vi "读取反控数据解析(子VI).vi"(6 "数据":string, 7 "命令编码CN":string) -> (2 "设置超时时间/min":i32=1, 3 "反控命令错误？":bool)   [LabVIEW 2016, in "数据传输系统.lvlib"]
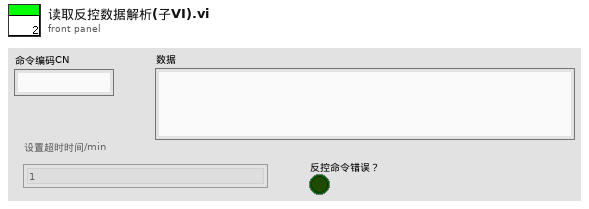
[diagram p1: front panel]
types:
  T1 = enum16{"初始化", "打开连接", "表格比对", "发送数据", "读取数据", "数据处理"}
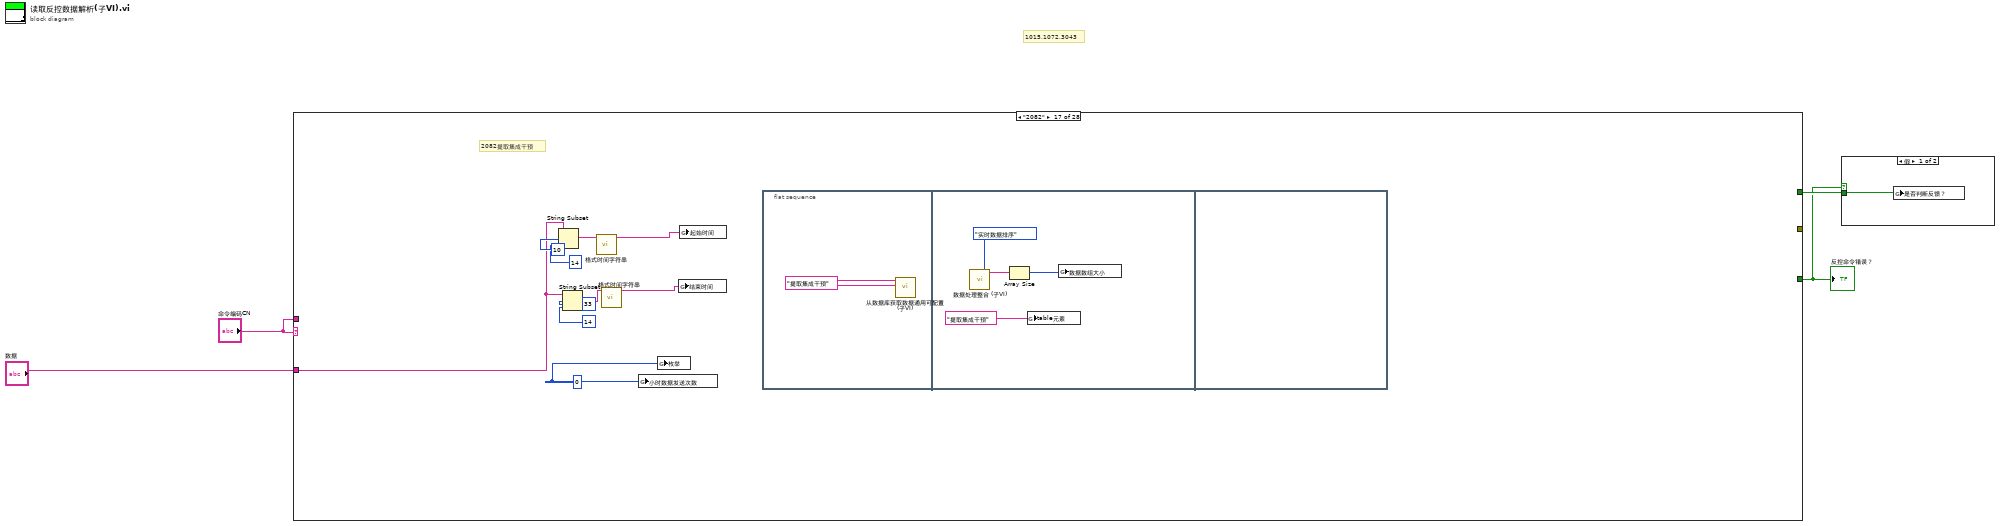
[diagram p0: block diagram]
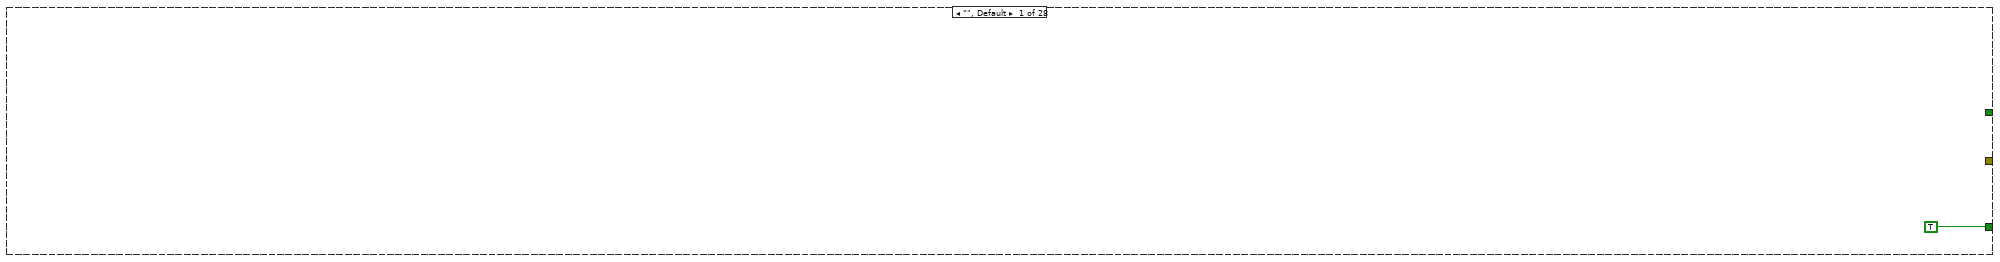
[diagram p3: hidden frame]
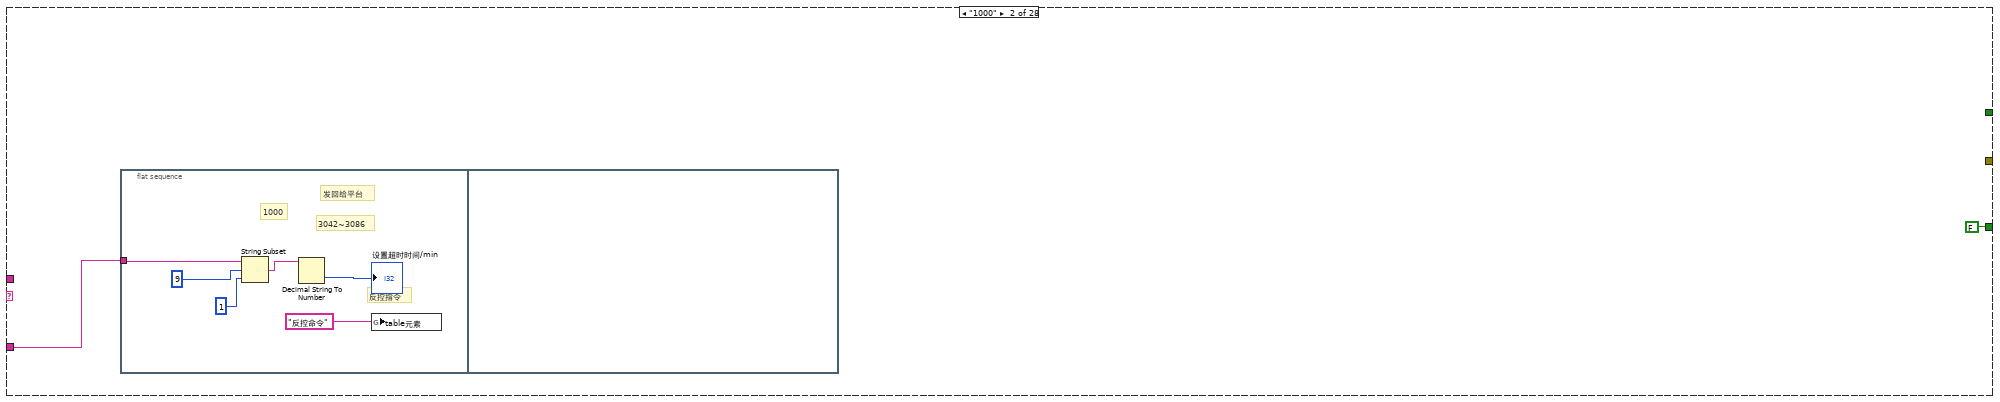
[diagram p4: hidden frame]
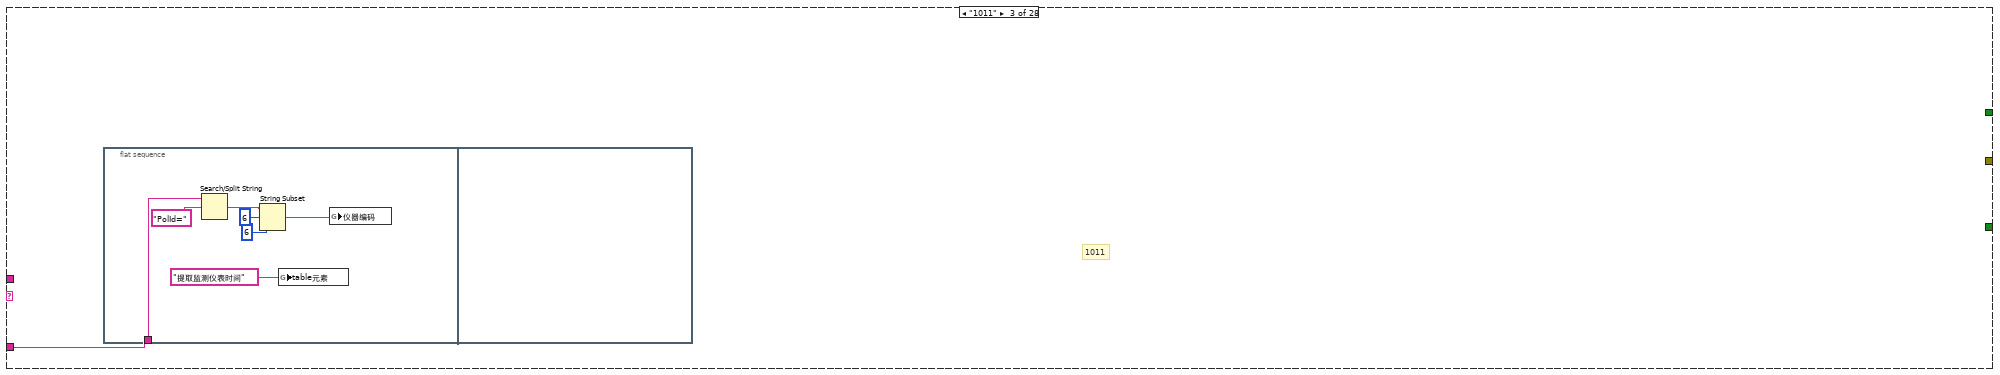
[diagram p5: hidden frame]
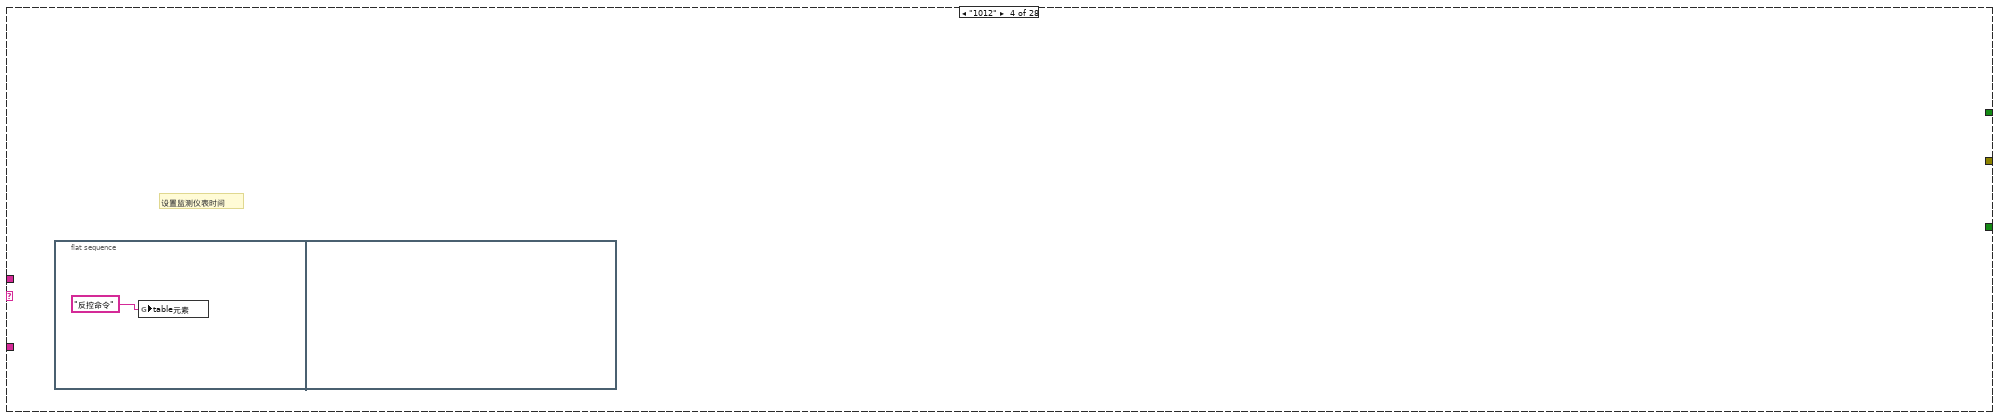
[diagram p6: hidden frame]
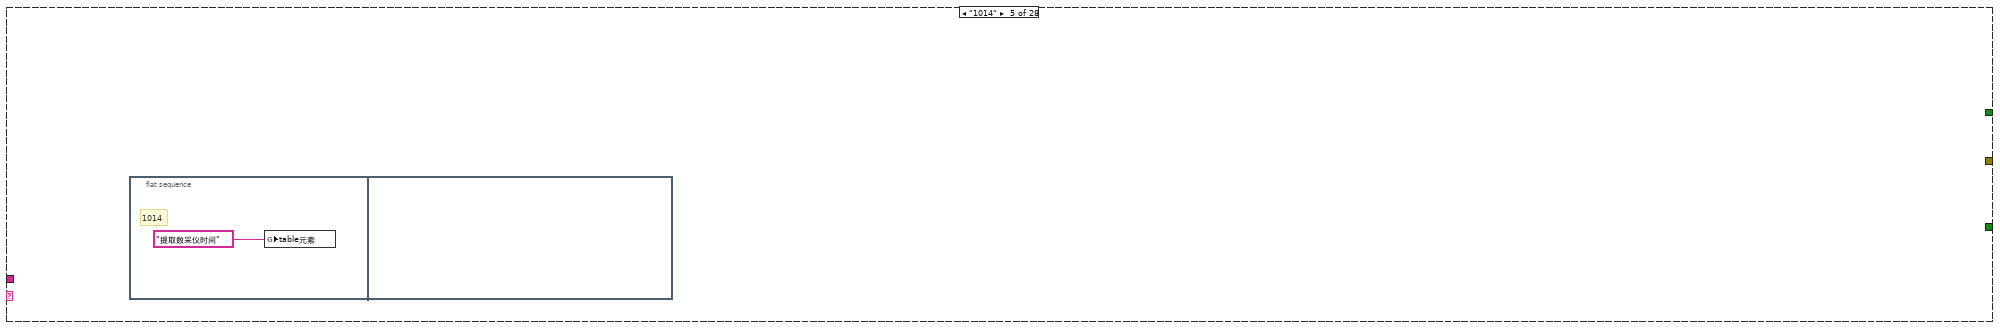
[diagram p7: hidden frame]
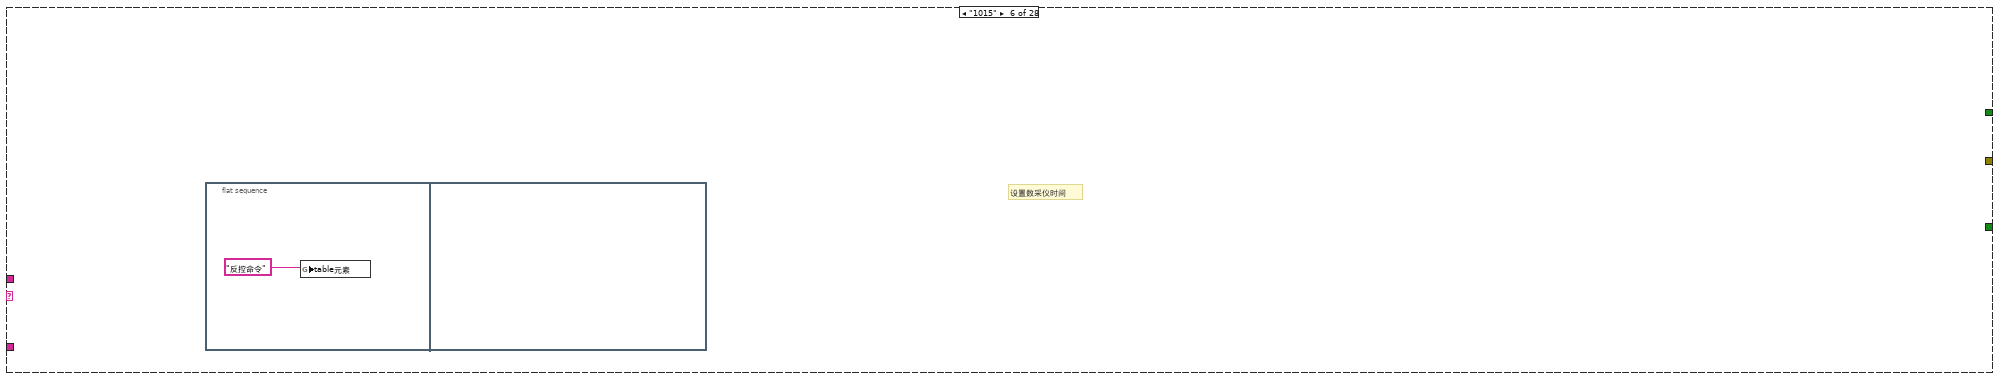
[diagram p8: hidden frame]
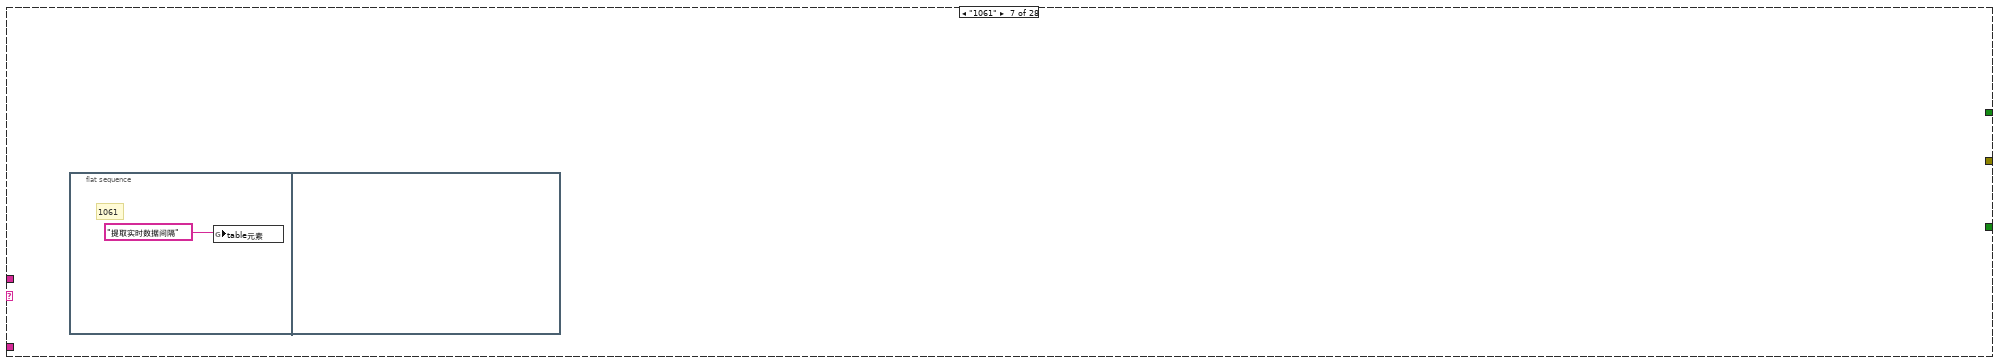
[diagram p9: hidden frame]
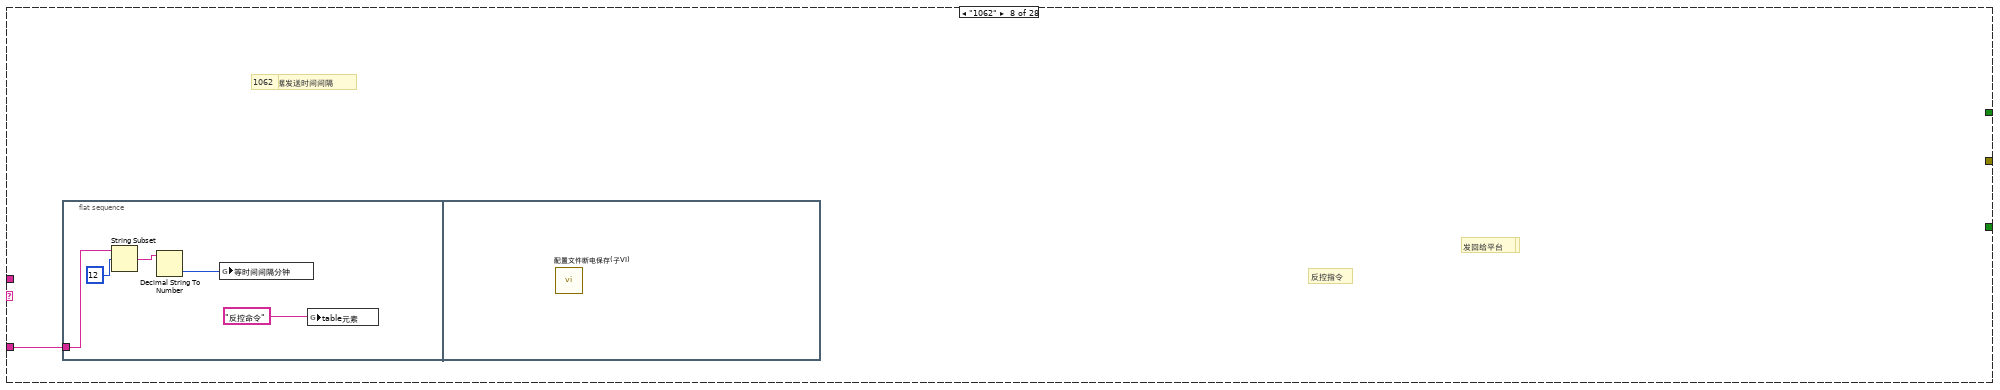
[diagram p10: hidden frame]
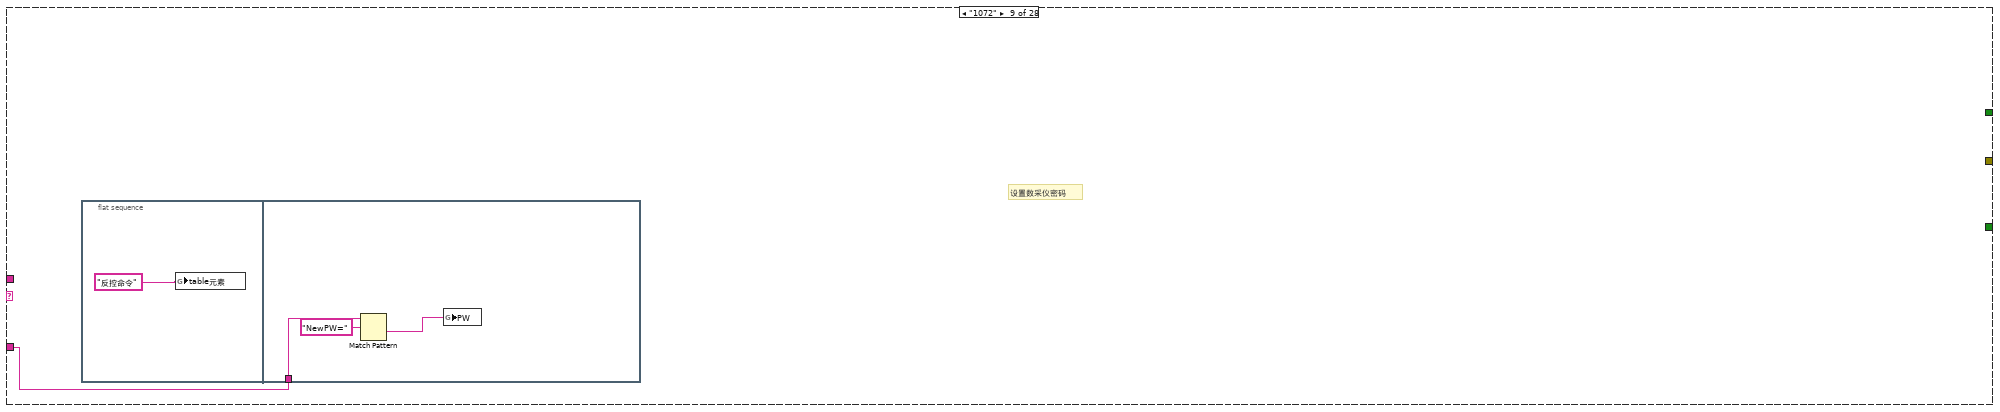
[diagram p11: hidden frame]
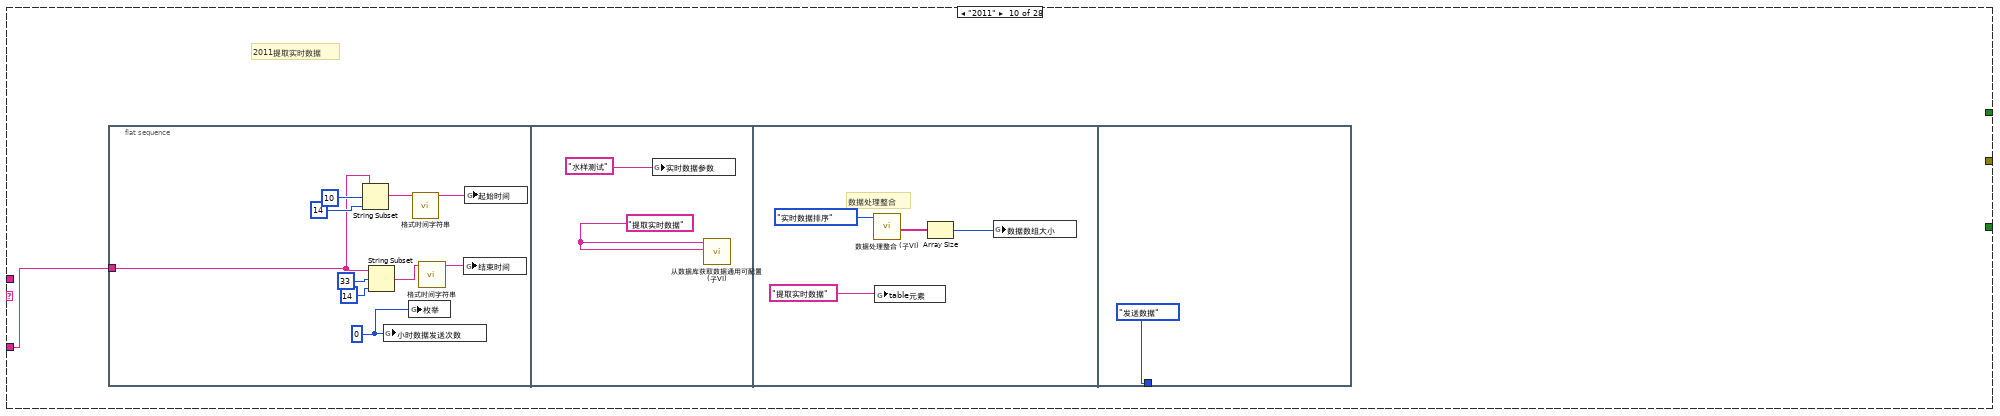
[diagram p12: hidden frame]
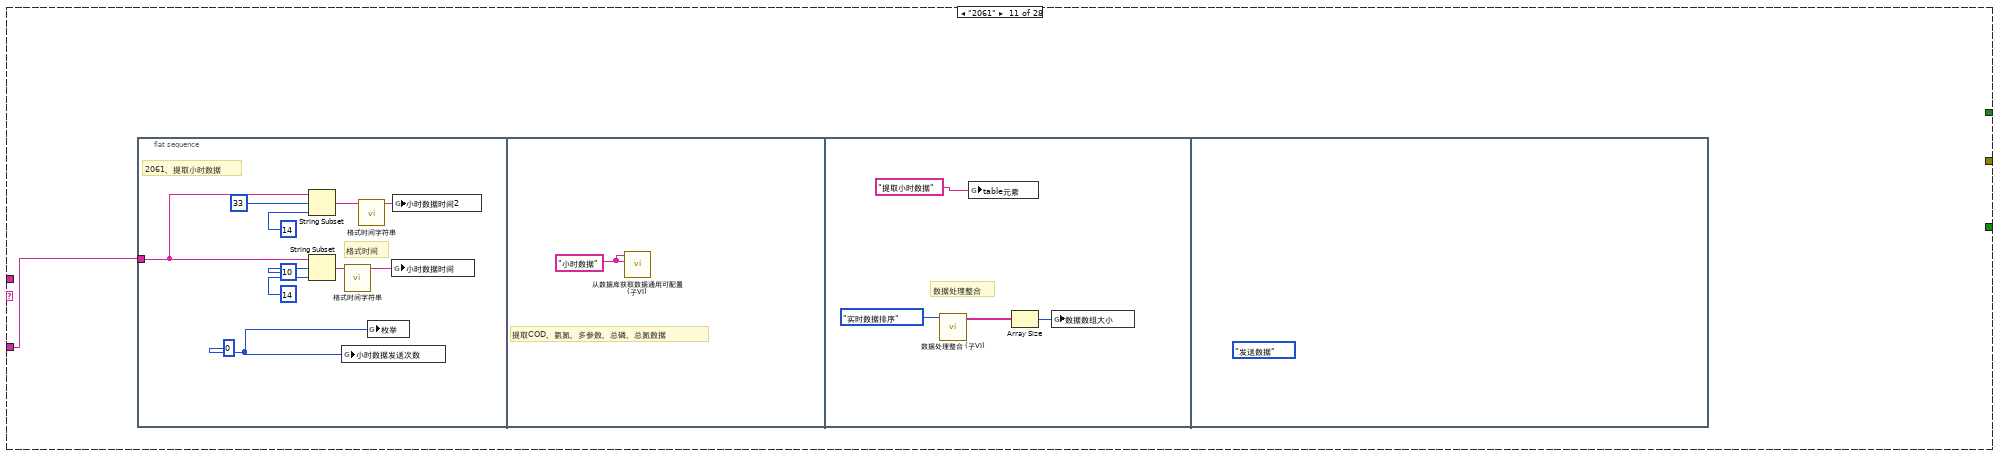
[diagram p13: hidden frame]
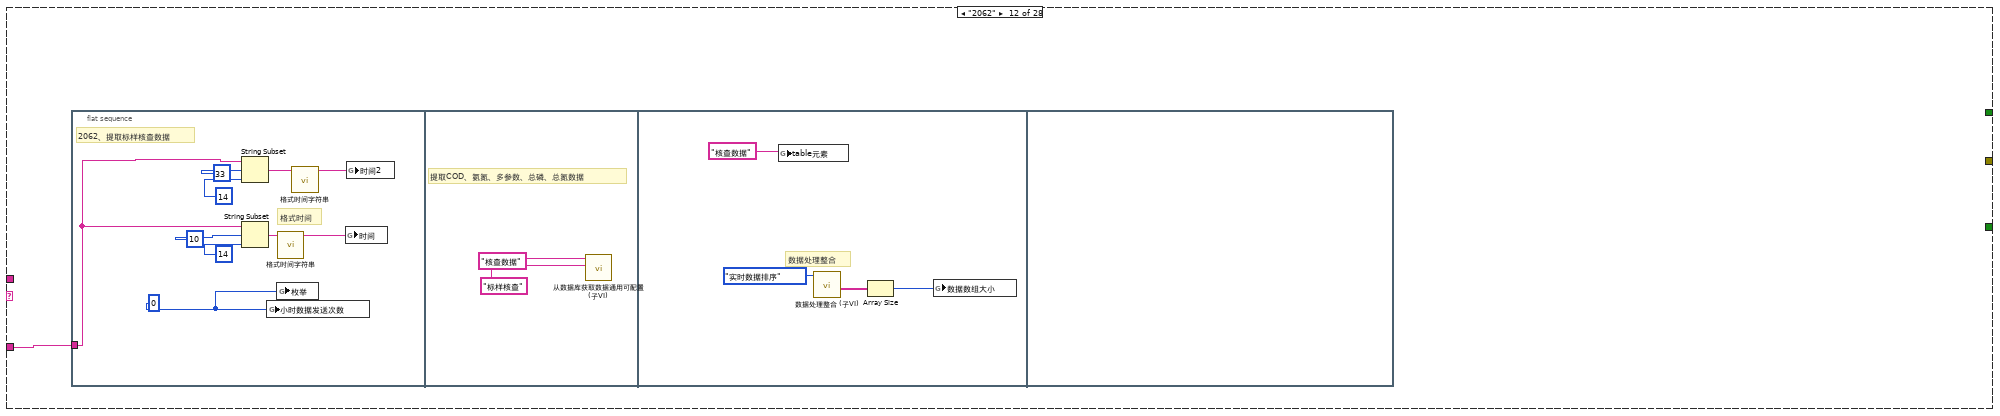
[diagram p14: hidden frame]
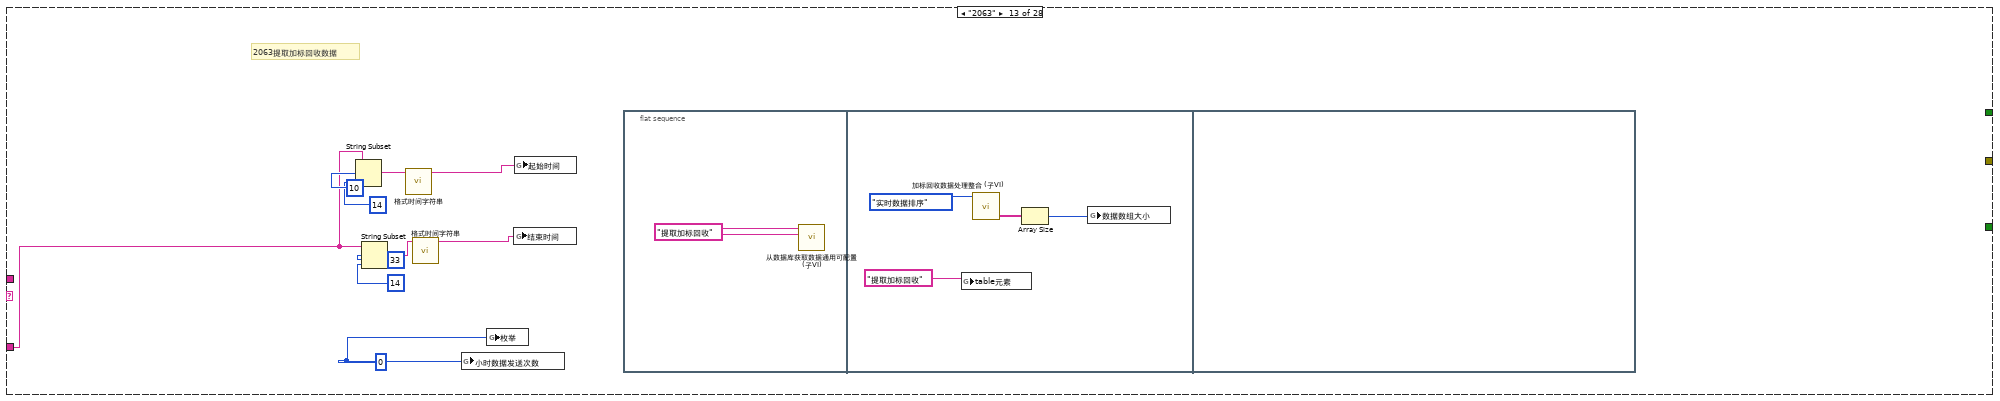
[diagram p15: hidden frame]
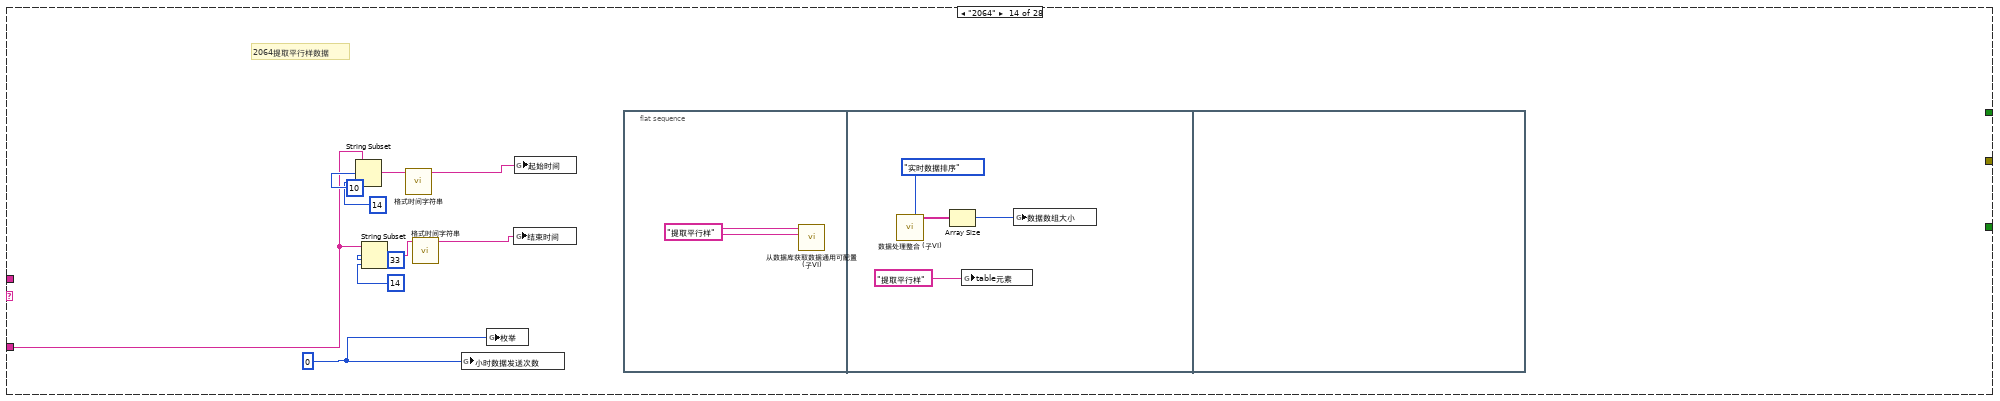
[diagram p16: hidden frame]
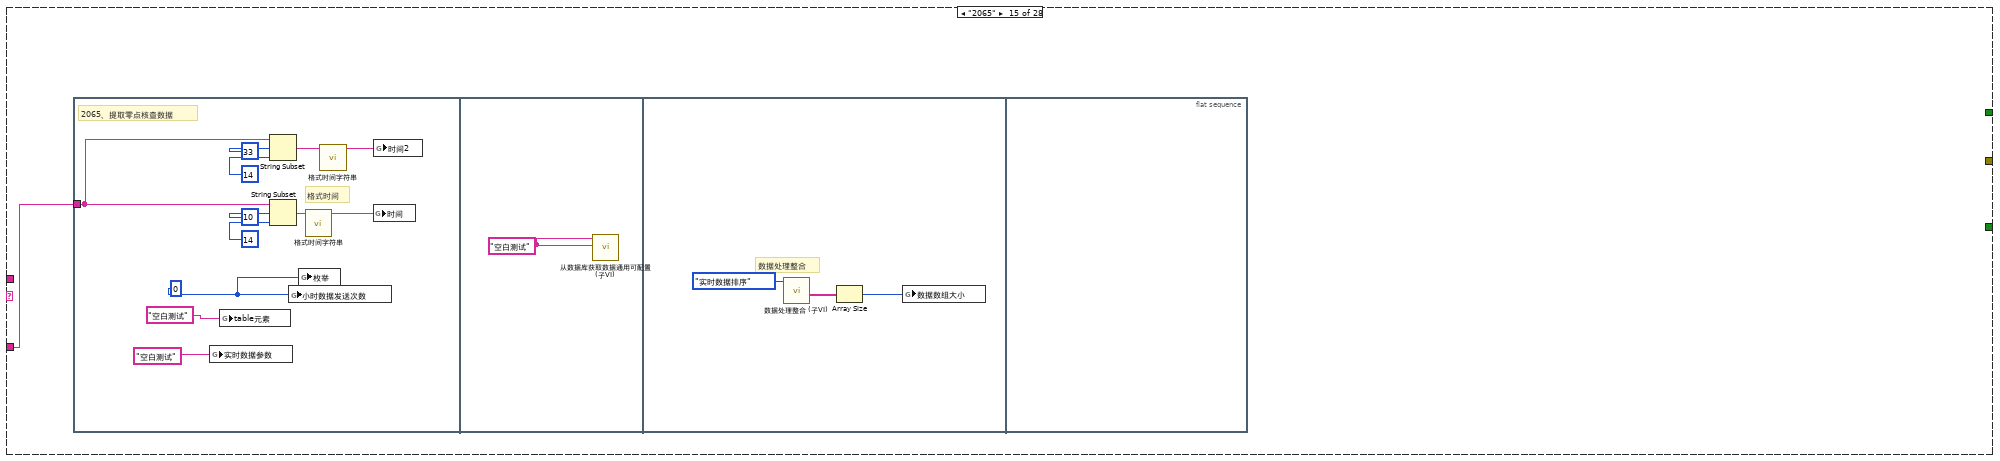
[diagram p17: hidden frame]
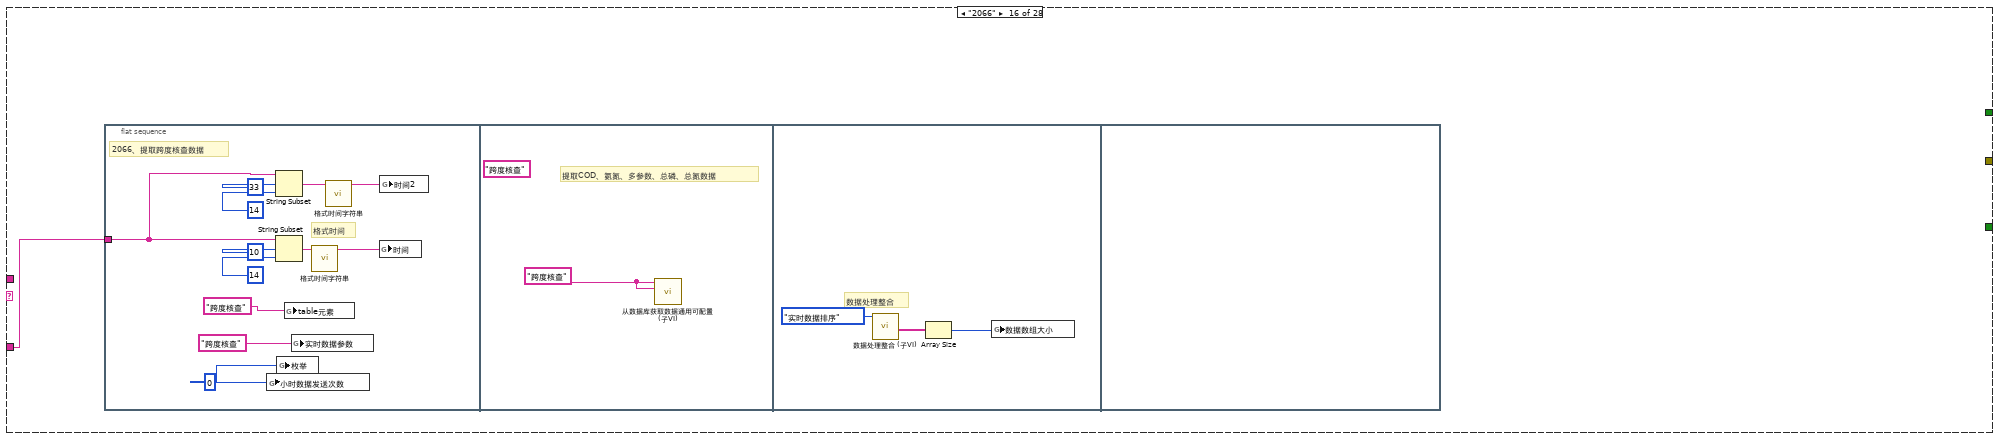
[diagram p18: hidden frame]
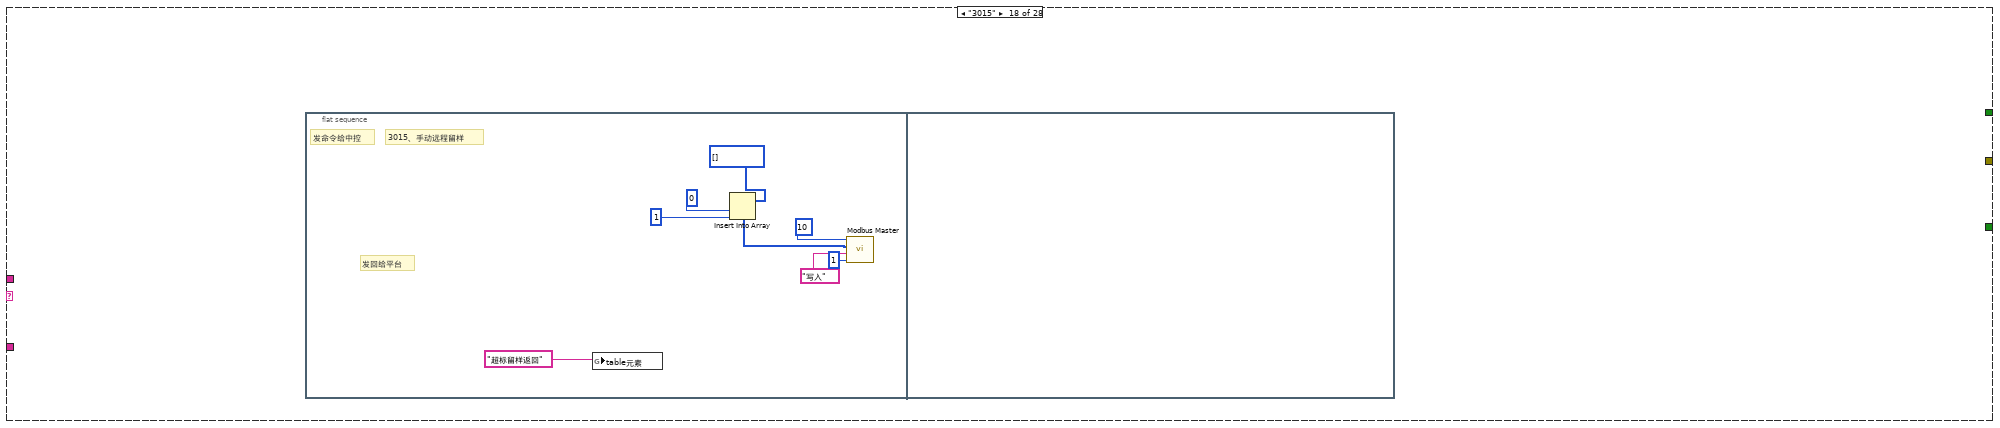
[diagram p19: hidden frame]
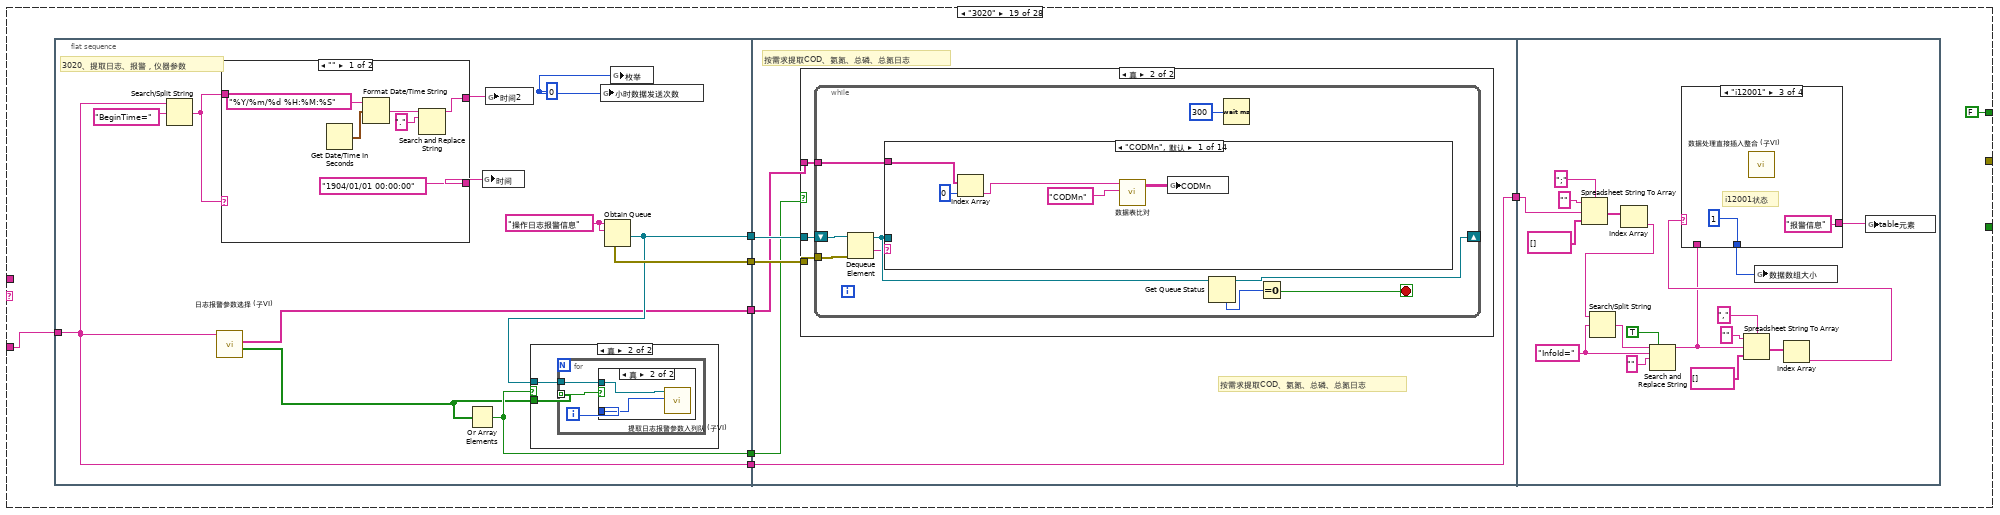
[diagram p20: hidden frame]
diagram:
  # "1015,1072,3043"
  n1 = case shown="\"2082\"" "命令编码CN" {
    tunnel: "命令编码CN" -> [_ _ _ _ _ _ _ _ _ _ _ _ _ _ _ _ _ _ _ _ _ _ _ _ _ _ _ w475]
    tunnel: "数据" -> [_ w7 w14 _ _ _ _ w26 w32 w37 w55 w71 w88 w103 w118 w135 w152 _ w178 w334 _ _ w412 _ _ _ w456 w472]
    tunnel: [_ _ _ _ _ _ _ _ _ _ _ _ _ _ _ _ _ _ _ _ _ _ _ _ _ _ _ w470] -> _
    tunnel: [TRUE FALSE _ _ _ _ _ _ _ _ _ _ _ _ _ _ _ _ _ _ _ _ _ _ _ _ _ _] -> w1
    tunnel: [_ _ _ _ _ _ _ _ _ _ _ _ _ _ _ _ _ _ FALSE ("是否判断反馈？") TRUE ("是否判断反馈？") _ _ TRUE ("是否判断反馈？") _ TRUE ("是否判断反馈？") TRUE ("是否判断反馈？") _ TRUE ("是否判断反馈？")] -> w2
    frame "", Default {
    }
    frame "1000" {
      n2 = flat-sequence {
        tunnel: w7 -> [w9]
        frame #0 {
          # "发回给平台"
          # "3042~3086"
          # "反控指令"
          # "1000"
          n3 = String Subset(string=w9, offset (0)=9 ("偏移量(0)"), length (rest)=1 ("长度（剩余）")) -> (substring=w11:string)
          n4 = Decimal String To Number(string=w11) -> (number=→"设置超时时间/min":i32)  [unwired: 2 in, 1 out]
          n5 = global write "全局1.vi" "table元素"("反控命令" ("新元素/子数组")) -> ()
        }
        frame #1 {
        }
      }
    }
    frame "1011" {
      # "1011"
      n6 = flat-sequence {
        tunnel: w14 -> [w16]
        frame #0 {
          n7 = Search/Split String(string=w16, search string/char (-)="PolId=" ("搜索字符串/字符(-)")) -> (match + rest of string=w20:string)  [unwired: 1 in, 2 out]
          n8 = String Subset(string=w20, offset (0)=6 ("偏移量(0)"), length (rest)=6 ("长度（剩余）")) -> (substring=w17:string)
          n9 = global write "全局1.vi" "table元素"("提取监测仪表时间") -> ()
          n10 = global write "全局 提取仪器参数.vi" "仪器编码"(w17) -> ()
        }
        frame #1 {
        }
      }
    }
    frame "1012" {
      # "设置监测仪表时间"
      n11 = flat-sequence {
        frame #0 {
          n12 = global write "全局1.vi" "table元素"("反控命令" ("新元素/子数组")) -> ()
        }
        frame #1 {
        }
      }
    }
    frame "1014" {
      n13 = flat-sequence {
        frame #0 {
          # "1014"
          n14 = global write "全局1.vi" "table元素"("提取数采仪时间") -> ()
        }
        frame #1 {
        }
      }
    }
    frame "1015" {
      # "设置数采仪时间"
      n15 = flat-sequence {
        frame #0 {
          n16 = global write "全局1.vi" "table元素"("反控命令" ("新元素/子数组")) -> ()
        }
        frame #1 {
        }
      }
    }
    frame "1061" {
      n17 = flat-sequence {
        frame #0 {
          # "1061"
          n18 = global write "全局1.vi" "table元素"("提取实时数据间隔") -> ()
        }
        frame #1 {
        }
      }
    }
    frame "1062" {
      # "发回给平台"
      # "反控指令"
      # "3042~3086"
      # "设置数据发送时间间隔"
      # "1062"
      n19 = flat-sequence {
        tunnel: w26 -> [w29]
        frame #0 {
          n20 = String Subset(string=w29, offset (0)=12 ("偏移量(0)")) -> (substring=w30:string)  [unwired: 1 in]
          n21 = Decimal String To Number(string=w30) -> (number=w27:i32)  [unwired: 2 in, 1 out]
          n22 = global write "断电保存全局.vi" "等时间间隔分钟"(w27) -> ()
          n23 = global write "全局1.vi" "table元素"("反控命令" ("新元素/子数组")) -> ()
        }
        frame #1 {
          n24 = call "配置文件断电保存(子VI).vi"() -> ()  [unwired: 12 in]
        }
      }
    }
    frame "1072" {
      # "设置数采仪密码"
      n25 = flat-sequence {
        tunnel: w32 -> [w36]
        frame #0 {
          n26 = global write "全局1.vi" "table元素"("反控命令" ("新元素/子数组")) -> ()
        }
        frame #1 {
          n27 = Match Pattern(string=w36, regular expression="NewPW=" ("正则表达式")) -> (after substring=w34:string)  [unwired: 1 in, 3 out]
          n28 = global write "断电保存全局.vi" "PW"(w34) -> ()
        }
      }
    }
    frame "2011" {
      # "2011提取实时数据"
      n29 = flat-sequence {
        tunnel: w37 -> [w38]
        tunnel: [T1."发送数据" ("元素")] -> _
        frame #0 {
          w43 = 0 ("数值")
          n30 = String Subset(string=w38, offset (0)=10 ("偏移量(0)"), length (rest)=14 ("长度（剩余）")) -> (substring=w46:string)
          n31 = String Subset(string=w38, offset (0)=33 ("偏移量(0)"), length (rest)=14 ("长度（剩余）")) -> (substring=w44:string)
          n32 = global write "全局 小时数据发送次数.vi" "小时数据发送次数"(w43) -> ()
          n33 = global write "全局1.vi" "枚举"(w43) -> ()
          n34 = call "格式时间字符串.vi"("字符串"=w46) -> ("连接的字符串"=w47:string)  [unwired: 10 in]
          n35 = call "格式时间字符串.vi"("字符串"=w44) -> ("连接的字符串"=w45:string)  [unwired: 10 in]
          n36 = global write "起始时间.vi" "结束时间"(w45) -> ()
          n37 = global write "起始时间.vi" "起始时间"(w47) -> ()
        }
        frame #1 {
          w48 = "提取实时数据" ("新元素/子数组")
          n38 = global write "全局 实时数据参数.vi" "实时数据参数"("水样测试") -> ()
          n39 = call "从数据库获取数据通用可配置(子VI).vi"("table输入"=w48, "列队名（唯一）"=w48) -> ()  [unwired: 8 in, 2 out]
        }
        frame #2 {
          # "数据处理整合"
          n40 = call "数据处理整合 (子VI).vi"("枚举"=enum16{"实时数据排序", "小时数据排序"}."实时数据排序") -> ("已排序的数组"=w52:string[])  [unwired: 10 in]
          n41 = global write "全局1.vi" "table元素"("提取实时数据" ("新元素/子数组")) -> ()
          n42 = Array Size(array=w52) -> (size(s)=w53:i32)
          n43 = global write "全局 数据数组大小.vi" "数据数组大小"(w53) -> ()
        }
        frame #3 {
        }
      }
    }
    frame "2061" {
      n44 = flat-sequence {
        tunnel: w55 -> [w56]
        frame #0 {
          w57 = 0 ("数值")
          # "格式时间"
          # "2061、提取小时数据"
          n45 = String Subset(string=w56, offset (0)=33 ("偏移量(0)"), length (rest)=14 ("长度（剩余）")) -> (substring=w59:string)
          n46 = String Subset(string=w56, offset (0)=10 ("偏移量(0)"), length (rest)=14 ("长度（剩余）")) -> (substring=w60:string)
          n47 = global write "全局 小时数据发送次数.vi" "小时数据发送次数"(w57) -> ()
          n48 = call "格式时间字符串.vi"("字符串"=w60) -> ("连接的字符串"=w61:string)  [unwired: 10 in]
          n49 = call "格式时间字符串.vi"("字符串"=w59) -> ("连接的字符串"=w58:string)  [unwired: 10 in]
          n50 = global write "全局1.vi" "枚举"(w57) -> ()
          n51 = global write "全局 水样时间.vi" "小时数据时间"(w61) -> ()
          n52 = global write "全局 时间2.vi" "小时数据时间2"(w58) -> ()
        }
        frame #1 {
          w66 = "小时数据" ("名称（未命名）")
          # "提取COD、氨氮、多参数、总磷、总氮数据"
          n53 = call "从数据库获取数据通用可配置(子VI).vi"("table输入"=w66, "列队名（唯一）"=w66) -> ()  [unwired: 8 in, 2 out]
        }
        frame #2 {
          # "数据处理整合"
          n54 = call "数据处理整合 (子VI).vi"("枚举"=enum16{"实时数据排序", "小时数据排序"}."实时数据排序") -> ("已排序的数组"=w70:string[])  [unwired: 10 in]
          n55 = global write "全局1.vi" "table元素"("提取小时数据" ("新元素/子数组")) -> ()
          n56 = Array Size(array=w70) -> (size(s)=w69:i32)
          n57 = global write "全局 数据数组大小.vi" "数据数组大小"(w69) -> ()
        }
        frame #3 {
          (unwired) T1."发送数据" ("元素")
        }
      }
    }
    frame "2062" {
      n58 = flat-sequence {
        tunnel: w71 -> [w72]
        frame #0 {
          w73 = 0 ("数值")
          # "格式时间"
          # "2062、提取标样核查数据"
          n59 = String Subset(string=w72, offset (0)=33 ("偏移量(0)"), length (rest)=14 ("长度（剩余）")) -> (substring=w75:string)
          n60 = String Subset(string=w72, offset (0)=10 ("偏移量(0)"), length (rest)=14 ("长度（剩余）")) -> (substring=w76:string)
          n61 = global write "全局 小时数据发送次数.vi" "小时数据发送次数"(w73) -> ()
          n62 = global write "全局1.vi" "枚举"(w73) -> ()
          n63 = call "格式时间字符串.vi"("字符串"=w76) -> ("连接的字符串"=w77:string)  [unwired: 10 in]
          n64 = call "格式时间字符串.vi"("字符串"=w75) -> ("连接的字符串"=w74:string)  [unwired: 10 in]
          n65 = global write "全局 水样时间.vi" "时间"(w77) -> ()
          n66 = global write "全局 时间2.vi" "时间2"(w74) -> ()
        }
        frame #1 {
          # "提取COD、氨氮、多参数、总磷、总氮数据"
          n67 = call "从数据库获取数据通用可配置(子VI).vi"("table输入"="标样核查" ("新元素/子数组"), "列队名（唯一）"="核查数据" ("新元素/子数组")) -> ()  [unwired: 8 in, 2 out]
        }
        frame #2 {
          # "数据处理整合"
          n68 = global write "全局1.vi" "table元素"("核查数据" ("新元素/子数组")) -> ()
          n69 = call "数据处理整合 (子VI).vi"("枚举"=enum16{"实时数据排序", "小时数据排序"}."实时数据排序") -> ("已排序的数组"=w86:string[])  [unwired: 10 in]
          n70 = Array Size(array=w86) -> (size(s)=w87:i32)
          n71 = global write "全局 数据数组大小.vi" "数据数组大小"(w87) -> ()
        }
        frame #3 {
        }
      }
    }
    frame "2063" {
      w93 = 0 ("数值")
      # "2063提取加标回收数据"
      n72 = String Subset(string=w88, offset (0)=10 ("偏移量(0)"), length (rest)=14 ("长度（剩余）")) -> (substring=w90:string)
      n73 = String Subset(string=w88, offset (0)=33 ("偏移量(0)"), length (rest)=14 ("长度（剩余）")) -> (substring=w92:string)
      n74 = call "格式时间字符串.vi"("字符串"=w90) -> ("连接的字符串"=w89:string)  [unwired: 10 in]
      n75 = call "格式时间字符串.vi"("字符串"=w92) -> ("连接的字符串"=w91:string)  [unwired: 10 in]
      n76 = global write "全局 小时数据发送次数.vi" "小时数据发送次数"(w93) -> ()
      n77 = global write "全局1.vi" "枚举"(w93) -> ()
      n78 = global write "起始时间.vi" "结束时间"(w91) -> ()
      n79 = global write "起始时间.vi" "起始时间"(w89) -> ()
      n80 = flat-sequence {
        frame #0 {
          w98 = "提取加标回收" ("新元素/子数组")
          n81 = call "从数据库获取数据通用可配置(子VI).vi"("table输入"=w98, "列队名（唯一）"=w98) -> ()  [unwired: 8 in, 2 out]
        }
        frame #1 {
          n82 = global write "全局1.vi" "table元素"("提取加标回收" ("新元素/子数组")) -> ()
          n83 = call "加标回收数据处理整合 (子VI).vi"("枚举"=enum16{"实时数据排序", "小时数据排序"}."实时数据排序") -> ("已排序的数组"=w100:string[])  [unwired: 10 in]
          n84 = Array Size(array=w100) -> (size(s)=w102:i32)
          n85 = global write "全局 数据数组大小.vi" "数据数组大小"(w102) -> ()
        }
        frame #2 {
        }
      }
    }
    frame "2064" {
      w108 = 0 ("数值")
      # "2064提取平行样数据"
      n86 = String Subset(string=w103, offset (0)=10 ("偏移量(0)"), length (rest)=14 ("长度（剩余）")) -> (substring=w105:string)
      n87 = String Subset(string=w103, offset (0)=33 ("偏移量(0)"), length (rest)=14 ("长度（剩余）")) -> (substring=w107:string)
      n88 = call "格式时间字符串.vi"("字符串"=w105) -> ("连接的字符串"=w104:string)  [unwired: 10 in]
      n89 = call "格式时间字符串.vi"("字符串"=w107) -> ("连接的字符串"=w106:string)  [unwired: 10 in]
      n90 = global write "全局 小时数据发送次数.vi" "小时数据发送次数"(w108) -> ()
      n91 = global write "全局1.vi" "枚举"(w108) -> ()
      n92 = global write "起始时间.vi" "结束时间"(w106) -> ()
      n93 = global write "起始时间.vi" "起始时间"(w104) -> ()
      n94 = flat-sequence {
        frame #0 {
          w113 = "提取平行样" ("新元素/子数组")
          n95 = call "从数据库获取数据通用可配置(子VI).vi"("table输入"=w113, "列队名（唯一）"=w113) -> ()  [unwired: 8 in, 2 out]
        }
        frame #1 {
          n96 = call "数据处理整合 (子VI).vi"("枚举"=enum16{"实时数据排序", "小时数据排序"}."实时数据排序") -> ("已排序的数组"=w117:string[])  [unwired: 10 in]
          n97 = Array Size(array=w117) -> (size(s)=w116:i32)
          n98 = global write "全局1.vi" "table元素"("提取平行样" ("新元素/子数组")) -> ()
          n99 = global write "全局 数据数组大小.vi" "数据数组大小"(w116) -> ()
        }
        frame #2 {
        }
      }
    }
    frame "2065" {
      n100 = flat-sequence {
        tunnel: w118 -> [w120]
        frame #0 {
          w121 = 0 ("数值")
          # "格式时间"
          # "2065、提取零点核查数据"
          n101 = global write "全局 实时数据参数.vi" "实时数据参数"("空白测试" ("新元素/子数组")) -> ()
          n102 = global write "全局1.vi" "table元素"("空白测试" ("新元素/子数组")) -> ()
          n103 = String Subset(string=w120, offset (0)=33 ("偏移量(0)"), length (rest)=14 ("长度（剩余）")) -> (substring=w124:string)
          n104 = String Subset(string=w120, offset (0)=10 ("偏移量(0)"), length (rest)=14 ("长度（剩余）")) -> (substring=w125:string)
          n105 = global write "全局 小时数据发送次数.vi" "小时数据发送次数"(w121) -> ()
          n106 = global write "全局1.vi" "枚举"(w121) -> ()
          n107 = call "格式时间字符串.vi"("字符串"=w125) -> ("连接的字符串"=w126:string)  [unwired: 10 in]
          n108 = call "格式时间字符串.vi"("字符串"=w124) -> ("连接的字符串"=w123:string)  [unwired: 10 in]
          n109 = global write "全局 水样时间.vi" "时间"(w126) -> ()
          n110 = global write "全局 时间2.vi" "时间2"(w123) -> ()
        }
        frame #1 {
          w131 = "空白测试" ("新元素/子数组")
          n111 = call "从数据库获取数据通用可配置(子VI).vi"("table输入"=w131, "列队名（唯一）"=w131) -> ()  [unwired: 8 in, 2 out]
        }
        frame #2 {
          # "数据处理整合"
          n112 = call "数据处理整合 (子VI).vi"("枚举"=enum16{"实时数据排序", "小时数据排序"}."实时数据排序") -> ("已排序的数组"=w133:string[])  [unwired: 10 in]
          n113 = Array Size(array=w133) -> (size(s)=w134:i32)
          n114 = global write "全局 数据数组大小.vi" "数据数组大小"(w134) -> ()
        }
        frame #3 {
        }
      }
    }
    frame "2066" {
      n115 = flat-sequence {
        tunnel: w135 -> [w137]
        frame #0 {
          w138 = 0 ("数值")
          # "格式时间"
          # "2066、提取跨度核查数据"
          n116 = global write "全局 小时数据发送次数.vi" "小时数据发送次数"(w138) -> ()
          n117 = String Subset(string=w137, offset (0)=33 ("偏移量(0)"), length (rest)=14 ("长度（剩余）")) -> (substring=w141:string)
          n118 = String Subset(string=w137, offset (0)=10 ("偏移量(0)"), length (rest)=14 ("长度（剩余）")) -> (substring=w142:string)
          n119 = global write "全局1.vi" "枚举"(w138) -> ()
          n120 = global write "全局1.vi" "table元素"("跨度核查" ("新元素/子数组")) -> ()
          n121 = global write "全局 实时数据参数.vi" "实时数据参数"("跨度核查" ("新元素/子数组")) -> ()
          n122 = call "格式时间字符串.vi"("字符串"=w142) -> ("连接的字符串"=w143:string)  [unwired: 10 in]
          n123 = call "格式时间字符串.vi"("字符串"=w141) -> ("连接的字符串"=w140:string)  [unwired: 10 in]
          n124 = global write "全局 水样时间.vi" "时间"(w143) -> ()
          n125 = global write "全局 时间2.vi" "时间2"(w140) -> ()
        }
        frame #1 {
          w148 = "跨度核查" ("新元素/子数组")
          (unwired) "跨度核查" ("名称（未命名）")
          # "提取COD、氨氮、多参数、总磷、总氮数据"
          n126 = call "从数据库获取数据通用可配置(子VI).vi"("table输入"=w148, "列队名（唯一）"=w148) -> ()  [unwired: 8 in, 2 out]
        }
        frame #2 {
          # "数据处理整合"
          n127 = call "数据处理整合 (子VI).vi"("枚举"=enum16{"实时数据排序", "小时数据排序"}."实时数据排序") -> ("已排序的数组"=w151:string[])  [unwired: 10 in]
          n128 = Array Size(array=w151) -> (size(s)=w150:i32)
          n129 = global write "全局 数据数组大小.vi" "数据数组大小"(w150) -> ()
        }
        frame #3 {
        }
      }
    }
    frame "2082" {
      w157 = 0 ("数值")
      # "2082提取集成干预"
      n130 = String Subset(string=w152, offset (0)=10 ("偏移量(0)"), length (rest)=14 ("长度（剩余）")) -> (substring=w154:string)
      n131 = String Subset(string=w152, offset (0)=33 ("偏移量(0)"), length (rest)=14 ("长度（剩余）")) -> (substring=w156:string)
      n132 = call "格式时间字符串.vi"("字符串"=w154) -> ("连接的字符串"=w153:string)  [unwired: 10 in]
      n133 = call "格式时间字符串.vi"("字符串"=w156) -> ("连接的字符串"=w155:string)  [unwired: 10 in]
      n134 = global write "全局 小时数据发送次数.vi" "小时数据发送次数"(w157) -> ()
      n135 = global write "全局1.vi" "枚举"(w157) -> ()
      n136 = global write "起始时间.vi" "结束时间"(w155) -> ()
      n137 = global write "起始时间.vi" "起始时间"(w153) -> ()
      n138 = flat-sequence {
        frame #0 {
          w162 = "提取集成干预" ("新元素/子数组")
          n139 = call "从数据库获取数据通用可配置(子VI).vi"("table输入"=w162, "列队名（唯一）"=w162) -> ()  [unwired: 8 in, 2 out]
        }
        frame #1 {
          n140 = call "数据处理整合 (子VI).vi"("枚举"=enum16{"实时数据排序", "小时数据排序"}."实时数据排序") -> ("已排序的数组"=w166:string[])  [unwired: 10 in]
          n141 = Array Size(array=w166) -> (size(s)=w165:i32)
          n142 = global write "全局1.vi" "table元素"("提取集成干预" ("新元素/子数组")) -> ()
          n143 = global write "全局 数据数组大小.vi" "数据数组大小"(w165) -> ()
        }
        frame #2 {
        }
      }
    }
    frame "3015" {
      n144 = flat-sequence {
        frame #0 {
          # "发命令给中控"
          # "发回给平台"
          # "3015、手动远程留样"
          n145 = global write "全局1.vi" "table元素"("超标留样返回" ("新元素/子数组")) -> ()
          n146 = Insert Into Array(array=u16[] [] ("holding register values"), index=0 ("索引"), new element=u16 1 ("新元素/子数组")) -> (w170:u16[])
          n147 = call "Modbus Master.vi"("Unit ID"=u8 1, "读取写入选择"="写入", "holding register values"=w170, "starting address"=u16 10) -> ()  [unwired: 6 in, 2 out]
        }
        frame #1 {
        }
      }
    }
    frame "3020" {
      n148 = flat-sequence {
        tunnel: [w188] -> w182
        tunnel: [w189] -> w181
        tunnel: [w185] -> w180
        tunnel: [w187] -> w179
        tunnel: w178 -> [w186]
        tunnel: [w186] -> w176
        tunnel: w182 -> [w221]
        tunnel: w181 -> [w220]
        tunnel: w180 -> [w219]
        tunnel: w179 -> [w218]
        tunnel: [w217] -> w177
        tunnel: w176 -> [w217]
        tunnel: w177 -> [w305]
        frame #0 {
          w183 = "操作日志报警信息" ("名称（未命名）")
          w192 = 0 ("数值")
          # "3020、提取日志、报警，仪器参数"
          n149 = Search/Split String(string=w186, search string/char (-)="BeginTime=" ("搜索字符串")) -> (match + rest of string=w191:string)  [unwired: 1 in, 2 out]
          n150 = call "日志报警参数选择 (子VI).vi"("String输入"=w186) -> ("输出boll数组"=w184:bool[], "输出char数组"=w185:string[])  [unwired: 7 in, 2 out]
          n151 = case shown="\"\"" w191 {
            tunnel: ["1904/01/01 00:00:00" w214] -> w194
            tunnel: w191 -> [_ w208]
            tunnel: [w202 w209] -> w190
            frame "" {
              n152 = Get Date/Time In Seconds() -> (seconds since 1Jan1904=w204:timestamp)
              n153 = Format Date/Time String(time format string (%c)="%Y/%m/%d %H:%M:%S" ("时间格式字符串(%c)"), seconds (now)=w204) -> (date/time string=w205:string)  [unwired: 1 in]
              n154 = Search and Replace String(input string=w205, search string="." ("搜索字符串")) -> (result string=w202:string)  [unwired: 6 in, 3 out]
            }
            frame "真", Default {
              # "格式时间"
              n155 = String Subset(string=w208, offset (0)=33 ("偏移量(0)"), length (rest)=14 ("长度（剩余）")) -> (substring=w212:string)
              n156 = String Subset(string=w208, offset (0)=10 ("偏移量(0)"), length (rest)=14 ("长度（剩余）")) -> (substring=w213:string)
              n157 = call "格式时间字符串.vi"("字符串"=w212) -> ("连接的字符串"=w209:string)  [unwired: 10 in]
              n158 = call "格式时间字符串.vi"("字符串"=w213) -> ("连接的字符串"=w214:string)  [unwired: 10 in]
            }
          }
          n159 = Or Array Elements(Boolean array=w184) -> (logical OR=w187:bool)
          n160 = global write "全局 水样时间.vi" "时间"(w194) -> ()
          n161 = global write "全局 时间2.vi" "时间2"(w190) -> ()
          n162 = global write "全局 小时数据发送次数.vi" "小时数据发送次数"(w192) -> ()
          n163 = Obtain Queue(name (unnamed)=w183, element data type=w183) -> (queue out=w188:refnum<queue>, error out=w189:errorcluster)  [unwired: 3 in, 1 out]
          n164 = case shown="真" w187 {
            tunnel: w188 -> [_ w196]
            tunnel: w184 -> [_ w195]
            frame False {
            }
            frame True {
              n165 = for {
                tunnel: w195 -> [w198] mode=indexing
                tunnel: w196 -> [w197]
                i -> [w199]
                n166 = case shown="真" w198 {
                  tunnel: w199 -> [_ w201]
                  tunnel: w197 -> [_ w200]
                  frame False {
                  }
                  frame True {
                    n167 = call "提取日志报警参数入列队 (子VI).vi"("索引"=w201, "队列输入"=w200) -> ()  [unwired: 10 in]
                  }
                }
              }
            }
          }
          n168 = global write "全局1.vi" "枚举"(w192) -> ()
        }
        frame #1 {
          # "按需求提取COD、氨氮、总磷、总氮日志"
          # "按需求提取COD、氨氮、总磷、总氮日志"
          n169 = case shown="真" w218 {
            tunnel: w220 -> [_ w224]
            tunnel: w221 -> [_ w223]
            tunnel: w219 -> [_ w222]
            frame False {
            }
            frame True {
              n170 = while {
                shift-right: [w225] -> _
                shift-left: w223 -> [w233]
                tunnel: w224 -> [w232]
                tunnel: w222 -> [w226]
                stop <- w229 stop-if-true
                n171 = Dequeue Element(queue=w233, error in (no error)=w232) -> (queue out=w231:refnum<queue>, element=w227:string)  [unwired: 1 in, 2 out]
                n172 = case shown="\"CODMn\", 默认" w227 {
                  tunnel: w231 -> [_ _ _ _ _ _ _ _ _ _ _ _ _ _]
                  tunnel: w226 -> [w235 w240 w245 w250 w255 w261 w264 w269 w274 w279 w284 w289 w294 w299]
                  frame "CODMn", Default {
                    n173 = Index Array(array=w235, index=0 ("索引")) -> (element=w234:string)
                    n174 = call "数据表比对.vi"("仪器日志参数"="CODMn" ("元素"), "table输入"=w234) -> ("待发送数据"=w237:string[][])  [unwired: 6 in, 3 out]
                    n175 = global write "全局 所有参数.vi" "CODMn"(w237) -> ()
                  }
                  frame "CODCr" {
                    n176 = Index Array(array=w240, index=1 ("索引")) -> (element=w239:string)
                    n177 = call "数据表比对.vi"("仪器日志参数"="CODCr" ("元素"), "table输入"=w239) -> ("待发送数据"=w242:string[][])  [unwired: 6 in, 3 out]
                    n178 = global write "全局 所有参数.vi" "CODCr"(w242) -> ()
                  }
                  frame "氨氮" {
                    n179 = Index Array(array=w245, index=2 ("索引")) -> (element=w244:string)
                    n180 = call "数据表比对.vi"("仪器日志参数"="氨氮" ("元素"), "table输入"=w244) -> ("待发送数据"=w247:string[][])  [unwired: 6 in, 3 out]
                    n181 = global write "全局 所有参数.vi" "氨氮"(w247) -> ()
                  }
                  frame "总磷" {
                    n182 = Index Array(array=w250, index=3 ("索引")) -> (element=w249:string)
                    n183 = call "数据表比对.vi"("仪器日志参数"="总磷" ("元素"), "table输入"=w249) -> ("待发送数据"=w252:string[][])  [unwired: 6 in, 3 out]
                    n184 = global write "全局 所有参数.vi" "总磷"(w252) -> ()
                  }
                  frame "总氮" {
                    n185 = Index Array(array=w255, index=4 ("索引")) -> (element=w254:string)
                    n186 = call "数据表比对.vi"("仪器日志参数"="总氮" ("元素"), "table输入"=w254) -> ("待发送数据"=w257:string[][])  [unwired: 6 in, 3 out]
                    n187 = global write "全局 所有参数.vi" "总氮"(w257) -> ()
                  }
                  frame "数采仪" {
                    n188 = Index Array(array=w261, index=5 ("索引")) -> (element=w259:string)
                    n189 = call "数据表比对.vi"("仪器日志参数"="系统" ("元素"), "table输入"=w259) -> ("待发送数据"=w262:string[][])  [unwired: 6 in, 3 out]
                    n190 = global write "全局 所有参数.vi" "DO"(w262) -> ()
                  }
                  frame "PH" {
                    n191 = Index Array(array=w264, index=6 ("索引")) -> (element=w265:string)
                    n192 = call "数据表比对.vi"("仪器日志参数"="PH" ("元素"), "table输入"=w265) -> ("待发送数据"=w267:string[][])  [unwired: 6 in, 3 out]
                    n193 = global write "全局 所有参数.vi" "PH"(w267) -> ()
                  }
                  frame "电导率" {
                    n194 = Index Array(array=w269, index=7 ("索引")) -> (element=w270:string)
                    n195 = call "数据表比对.vi"("仪器日志参数"="电导率" ("元素"), "table输入"=w270) -> ("待发送数据"=w272:string[][])  [unwired: 6 in, 3 out]
                    n196 = global write "全局 所有参数.vi" "电导率"(w272) -> ()
                  }
                  frame "水温" {
                    n197 = Index Array(array=w274, index=8 ("索引")) -> (element=w275:string)
                    n198 = call "数据表比对.vi"("仪器日志参数"="水温" ("元素"), "table输入"=w275) -> ("待发送数据"=w277:string[][])  [unwired: 6 in, 3 out]
                    n199 = global write "全局 所有参数.vi" "水温"(w277) -> ()
                  }
                  frame "DO" {
                    n200 = Index Array(array=w279, index=9 ("索引")) -> (element=w280:string)
                    n201 = call "数据表比对.vi"("仪器日志参数"="溶解氧" ("元素"), "table输入"=w280) -> ("待发送数据"=w282:string[][])  [unwired: 6 in, 3 out]
                    n202 = global write "全局 所有参数.vi" "DO"(w282) -> ()
                  }
                  frame "浊度" {
                    n203 = Index Array(array=w284, index=10 ("索引")) -> (element=w285:string)
                    n204 = call "数据表比对.vi"("仪器日志参数"="浊度" ("元素"), "table输入"=w285) -> ("待发送数据"=w287:string[][])  [unwired: 6 in, 3 out]
                    n205 = global write "全局 所有参数.vi" "浊度"(w287) -> ()
                  }
                  frame "叶绿素" {
                    n206 = Index Array(array=w289, index=11 ("索引")) -> (element=w290:string)
                    n207 = call "数据表比对.vi"("仪器日志参数"="叶绿素" ("元素"), "table输入"=w290) -> ("待发送数据"=w292:string[][])  [unwired: 6 in, 3 out]
                    n208 = global write "全局 所有参数.vi" "叶绿素"(w292) -> ()
                  }
                  frame "藻密度" {
                    n209 = Index Array(array=w294, index=12 ("索引")) -> (element=w295:string)
                    n210 = call "数据表比对.vi"("仪器日志参数"="藻密度" ("元素"), "table输入"=w295) -> ("待发送数据"=w297:string[][])  [unwired: 6 in, 3 out]
                    n211 = global write "全局 所有参数.vi" "藻密度"(w297) -> ()
                  }
                  frame "ORP" {
                    n212 = Index Array(array=w299, index=13 ("索引")) -> (element=w300:string)
                    n213 = call "数据表比对.vi"("仪器日志参数"="ORP" ("元素"), "table输入"=w300) -> ("待发送数据"=w302:string[][])  [unwired: 6 in, 3 out]
                    n214 = global write "全局 所有参数.vi" "ORP"(w302) -> ()
                  }
                }
                n215 = Get Queue Status(queue=w231) -> (queue out=w225:refnum<queue>, # elements in queue=w230:i32)  [unwired: 2 in, 6 out]
                n216 = Wait (ms)(milliseconds to wait=u32 300 ("等待时间（毫秒）")) -> ()  [unwired: 1 out]
                n217 = Equal To 0?(x=w230) -> (x = 0?=w229:bool)
              }
            }
          }
        }
        frame #2 {
          w314 = "InfoId=" ("搜索字符串/字符(-)")
          n218 = Spreadsheet String To Array(delimiter (Tab)=";" ("分隔符(Tab)"), format string="" ("格式字符串"), spreadsheet string=w305, array type (2D Dbl)=string[] []) -> (array=w306:string[])
          n219 = Index Array(array=w306) -> (element=w304:string)  [unwired: 1 in]
          n220 = Search/Split String(string=w304, search string/char (-)=w314) -> (match + rest of string=w313:string)  [unwired: 1 in, 2 out]
          n221 = Search and Replace String(replace all?=TRUE ("替换全部？(F)"), input string=w313, search string=w314, replace string="" ("替换字符串(\"\")")) -> (result string=w310:string)  [unwired: 4 in, 3 out]
          n222 = Spreadsheet String To Array(delimiter (Tab)="," ("分隔符(Tab)"), format string="" ("格式字符串"), spreadsheet string=w310, array type (2D Dbl)=string[] []) -> (array=w312:string[])
          n223 = Index Array(array=w312) -> (element=w311:string)  [unwired: 1 in]
          n224 = case shown="\"i12001\"" w311 {
            tunnel: ["操作日志" ("名称（未命名）") "提取仪器参数" ("名称（未命名）") "报警信息" ("名称（未命名）") "" ("名称（未命名）")] -> w320
            tunnel: [w322 1 ("数据数组大小") 1 _] -> w321
            tunnel: w310 -> [_ w326 _ _]
            frame "i11001", "i21001" {
              # "数据处理整合"
              # "i11001日志"
              n225 = call "数据处理整合 (子VI).vi"("枚举"=enum16{"实时数据排序", "小时数据排序"}."实时数据排序") -> ("已排序的数组"=w323:string[])  [unwired: 10 in]
              n226 = Array Size(array=w323) -> (size(s)=w322:i32)
            }
            frame "i13001", "i13002", "i13003", "i13004", "i13005", "i13006", "i13007", "i13008", "i13009", "i13010", "i13011", "i13012", "i13013", "i13014", "i13015", "i13016", "i13017", "i13101", "i13102", "i13103", "i13104", "i13105", "i13106", "i13107", "i13108", "i13109", "i13110" {
              n227 = global write "全局 提取仪器参数.vi" "参数编码"(w326) -> ()
              n228 = call "数据处理直接插入整合 (子VI).vi"() -> ()  [unwired: 12 in]
            }
            frame "i12001" {
              # "i12001状态"
              n229 = call "数据处理直接插入整合 (子VI).vi"() -> ()  [unwired: 12 in]
            }
            frame Default {
            }
          }
          n230 = global write "全局 数据数组大小.vi" "数据数组大小"(w321) -> ()
          n231 = global write "全局1.vi" "table元素"(w320) -> ()
        }
      }
    }
    frame "3021" {
      (unwired) u16 256 ("starting address")
      (unwired) "PolId=w01018,InfoId=i13004,i13004-Info=168.0"
      # "0: 无\n1: CODMn\n2: PH\n3: 氨氮\n4: 总氮\n5: 总磷\n6:CODCr\n7:电导率\n8:水温\n9:溶解氧\n10:浊度\n11:叶绿素\n12:藻密度\n13:ORP"
      # "设置仪器参数"
      n232 = call "设置仪器参数命令解析.vi"("String输入"=w334) -> ("设置参数信息数组"=w333:string[][])  [unwired: 9 in, 1 out]
      n233 = for {
        tunnel: w333 -> [w337] mode=indexing
        # "同时设置几个参数?"
        n234 = flat-sequence {
          tunnel: w337 -> [w347]
          tunnel: [w338] -> w335
          tunnel: [w399] -> w336
          tunnel: w335 -> [w399]
          tunnel: w336 -> [w403]
          frame #0 {
            # "设置仪表参数"
            # "3|4个字节"
            # "反控指令"
            # "发命令给中控"
            # "1.因子编码\n2.关键参数\n3.值"
            n235 = Index Array(array=w347) -> (element #1=w346:string, element #2=w343:string, element #3=w342:string)  [unwired: 3 in]
            n236 = case shown="\"i13006\", \"i13013\"" w343 {
              tunnel: w342 -> [w351 w356]
              tunnel: [w349 w352] -> w340
              frame "假", Default {
                n237 = Fract/Exp String To Number(string=w351) -> (number=w348:dbl)  [unwired: 3 in, 1 out]
                n238 = Build Array(w348) -> (w350:dbl[])
                n239 = call "FloatToHex.vi"("浮点数"=w350) -> ("DCBA整形输出"=w349:u16[])  [unwired: 10 in]
              }
              frame "i13006", "i13013" {
                n240 = call "格式时间字符串.vi"("字符串"=w356) -> ("连接的字符串"=w355:string)  [unwired: 10 in]
                n241 = call "日期字符串格式至时间格式转换(子VI).vi"("data[0]"=w355) -> ("time stamp"=w354:timestamp)  [unwired: 10 in]
                n242 = Build Array(w354) -> (w353:timestamp[])
                n243 = call "DateToHex.vi"("DATE"=w353) -> ("数组"=w352:u16[])  [unwired: 10 in]
              }
            }
            n244 = case shown="\"w01100\"" w346 {
              tunnel: [u16 0 ("starting address") u16 1 ("starting address") u16 2 ("starting address") u16 3 ("starting address") u16 4 ("starting address") u16 5 ("starting address") u16 6 ("starting address") u16 7 ("starting address") u16 8 ("starting address") u16 9 ("starting address") u16 10 ("starting address") u16 11 ("starting address") u16 12 ("starting address") u16 13 ("starting address")] -> w341
              frame "", Default {
              }
              frame "w01019" {
              }
              frame "w01001" {
              }
              frame "w21003" {
              }
              frame "w21001" {
              }
              frame "w21011" {
              }
              frame "w01018" {
              }
              frame "w01014" {
              }
              frame "w01010" {
              }
              frame "w01009" {
              }
              frame "w01003" {
              }
              frame "w01016" {
              }
              frame "w19011" {
              }
              frame "w01100" {
              }
            }
            n245 = case shown="\"i13013\"" w343 {
              tunnel: [u16 256 ("starting address") u16 256 ("starting address") u16 260 ("starting address") u16 264 ("starting address") u16 268 ("starting address") u16 272 ("starting address") u16 276 ("starting address") u16 280 ("starting address") u16 284 ("starting address") u16 288 ("starting address") u16 292 ("starting address") u16 296 ("starting address") u16 300 ("starting address") u16 304 ("starting address") u16 308 ("starting address") u16 312 ("starting address") u16 316 ("starting address") u16 320 ("starting address") u16 356 ("starting address") u16 360 ("starting address") u16 364 ("starting address") u16 368 ("starting address") u16 372 ("starting address") u16 376 ("starting address") u16 380 ("starting address") u16 384 ("starting address") u16 388 ("starting address") u16 392 ("starting address")] -> w338
              frame "", Default {
              }
              frame "i13001" {
              }
              frame "i13002" {
              }
              frame "i13003" {
              }
              frame "i13004" {
              }
              frame "i13005" {
              }
              frame "i13006" {
              }
              frame "i13007" {
              }
              frame "i13008" {
              }
              frame "i13009" {
              }
              frame "i13010" {
              }
              frame "i13011" {
              }
              frame "i13012" {
              }
              frame "i13013" {
              }
              frame "i13014" {
              }
              frame "i13015" {
              }
              frame "i13016" {
              }
              frame "i13017" {
              }
              frame "i13101" {
              }
              frame "i13102" {
              }
              frame "i13103" {
              }
              frame "i13104" {
              }
              frame "i13105" {
              }
              frame "i13106" {
              }
              frame "i13107" {
              }
              frame "i13108" {
              }
              frame "i13109" {
              }
              frame "i13110" {
              }
            }
            n246 = Build Array (concatenate)(w341, w340) -> (w339:u16[])
            n247 = call "Modbus Master.vi"("Unit ID"=u8 1, "读取写入选择"="写入", "holding register values"=w339, "starting address"=w338) -> ()  [unwired: 6 in, 2 out]
          }
          frame #1 {
            n248 = Wait (ms)(milliseconds to wait=u32 3000 ("等待时间（毫秒）")) -> ()  [unwired: 1 out]
          }
          frame #2 {
            n249 = global write "全局1.vi" "table元素"("反控命令" ("新元素/子数组")) -> ()
            n250 = call "Modbus Master.vi"("Unit ID"=u8 1, "读取写入选择"="写入", "holding register values"=u16[] [0], "starting address"=w403) -> ()  [unwired: 6 in, 2 out]
          }
        }
      }
    }
    frame "3040" {
      # "提取现场系统信息（3040）"
      n251 = flat-sequence {
        frame #0 {
          n252 = global write "全局1.vi" "table元素"("提取现场系统信息" ("新元素/子数组")) -> ()
        }
        frame #1 {
        }
      }
    }
    frame "3041" {
      # "提取现场经纬度及环境信息（3041）"
      n253 = flat-sequence {
        frame #0 {
          n254 = global write "全局1.vi" "table元素"("提取经纬度环境信息" ("新元素/子数组")) -> ()
          n255 = call "数据表比对.vi"("table输入"="环境参数" ("新元素/子数组")) -> ("columns输出"=w407:string[], "待发送数据"=w409:string[][])  [unwired: 7 in, 2 out]
          n256 = global write "全局 环境参数.vi" "columns输出"(w407) -> ()
          n257 = global write "全局 环境参数.vi" "环境参数"(w409) -> ()
        }
        frame #1 {
        }
      }
    }
    frame "3042" {
      n258 = flat-sequence {
        tunnel: w412 -> [w414]
        frame #0 {
          # "反控指令"
          # "反控指令\n切换运行模式"
          # "发命令给中控"
          # "0维护，1常规，2应急，3质控"
          n259 = Search/Split String(string=w414, search string/char (-)="RunMode" ("搜索字符串/字符(-)")) -> (match + rest of string=w425:string)  [unwired: 1 in, 2 out]
          n260 = String Subset(string=w425, offset (0)=8 ("偏移量(0)"), length (rest)=1 ("长度（剩余）")) -> (substring=w422:string)
          n261 = case shown="\"0\", 默认" w422 {
            tunnel: [u16 0 ("新元素/子数组") u16 1 ("新元素/子数组") u16 2 ("新元素/子数组") u16 3 ("新元素/子数组")] -> w418
            frame "0", Default {
            }
            frame "1" {
            }
            frame "2" {
            }
            frame "3" {
            }
          }
          n262 = global write "全局1.vi" "table元素"("反控命令" ("新元素/子数组")) -> ()
          n263 = Insert Into Array(array=u16[] [] ("holding register values"), index=0 ("索引"), new element=w418) -> (w419:u16[])
          n264 = call "Modbus Master.vi"("Unit ID"=u8 1, "读取写入选择"="写入", "holding register values"=w419, "starting address"=u16 0) -> ()  [unwired: 6 in, 2 out]
        }
        frame #1 {
        }
      }
    }
    frame "3043" {
      # "远程重启工控机"
      n265 = flat-sequence {
        frame #0 {
          n266 = global write "全局1.vi" "table元素"("反控命令" ("新元素/子数组")) -> ()
        }
        frame #1 {
          n267 = call <vilib>:"System Exec.vi"("command line"="cmd /c shutdown/r") -> ("error out"=w432:errorcluster)  [unwired: 7 in, 3 out]
          n268 = call <vilib>:"Clear Errors.vi"("error in (no error)"=w432) -> ()  [unwired: 5 in, 2 out]
        }
      }
    }
    frame "3044" {
      n269 = flat-sequence {
        frame #0 {
          # "反控指令"
          # "发命令给中控"
          n270 = call "Modbus Master.vi"("Unit ID"=u8 1, "读取写入选择"="写入", "holding register values"=u16[] [1], "starting address"=u16 2) -> ()  [unwired: 6 in, 2 out]
        }
        frame #1 {
          # "反控指令\n单次测量"
          n271 = Wait (ms)(milliseconds to wait=u32 3000 ("等待时间（毫秒）")) -> ()  [unwired: 1 out]
        }
        frame #2 {
          n272 = global write "全局1.vi" "table元素"("反控命令" ("新元素/子数组")) -> ()
          n273 = call "Modbus Master.vi"("Unit ID"=u8 1, "读取写入选择"="写入", "holding register values"=u16[] [0], "starting address"=u16 2) -> ()  [unwired: 6 in, 2 out]
        }
      }
    }
    frame "3045", "3046" {
      n274 = flat-sequence {
        frame #0 {
          # "发命令给中控"
          n275 = call "Modbus Master.vi"("Unit ID"=u8 1, "读取写入选择"="写入", "holding register values"=u16[] [1], "starting address"=u16 3) -> ()  [unwired: 6 in, 2 out]
        }
        frame #1 {
          # "反控指令"
          # "反控指令\n急停"
          # "3045"
          n276 = Wait (ms)(milliseconds to wait=u32 3000 ("等待时间（毫秒）")) -> ()  [unwired: 1 out]
        }
        frame #2 {
          n277 = global write "全局1.vi" "table元素"("反控命令" ("新元素/子数组")) -> ()
          n278 = call "Modbus Master.vi"("Unit ID"=u8 1, "读取写入选择"="写入", "holding register values"=u16[] [0], "starting address"=u16 3) -> ()  [unwired: 6 in, 2 out]
        }
        frame #3 {
        }
      }
    }
    frame "3056" {
      n279 = flat-sequence {
        tunnel: w456 -> [w458]
        frame #0 {
          # "发回给平台"
          # "设置测量时间间隔"
          # "发命令给中控"
          n280 = Search/Split String(string=w458, search string/char (-)="RunInterval" ("搜索字符串/字符(-)")) -> (match + rest of string=w465:string)  [unwired: 1 in, 2 out]
          n281 = Decimal String To Number(string=w465, offset=12 ("偏移量(0)")) -> (number=w461:i32)  [unwired: 1 in, 1 out]
          n282 = Insert Into Array(array=u16[] [] ("holding register values"), index=0 ("索引"), new element=w461) -> (w460:u16[])
          n283 = global write "全局1.vi" "table元素"("反控命令" ("新元素/子数组")) -> ()
          n284 = call "Modbus Master.vi"("Unit ID"=u8 1, "读取写入选择"="写入", "holding register values"=w460, "starting address"=u16 14) -> ()  [unwired: 6 in, 2 out]
        }
        frame #1 {
        }
      }
    }
    frame "3080", "3081", "3082", "3083", "3084", "3085", "3086" {
      n285 = flat-sequence {
        tunnel: w475 -> [w479]
        tunnel: [w477] -> w474
        tunnel: w472 -> [w476]
        tunnel: w474 -> [w504]
        tunnel: [w504] -> w473
        tunnel: w473 -> [w509]
        tunnel: [w506] -> w471
        tunnel: [w512] -> w470
        tunnel: w471 -> [w512]
        frame #0 {
          # "30 启动标液核查  1CODmn  2 氨氮  3总磷  4总氮  5CODCr\n31 加标回收\n32 平行样测试\n33 零点核查\n34 跨度核查\n35 校零\n36 校标"
          # "1CODmn  2 氨氮  3总磷  4总氮  5CODCr"
          # "启动单台仪器标液核查"
          # "发命令给中控"
          n286 = Search/Split String(string=w476, search string/char (-)="PolId" ("搜索字符串/字符(-)")) -> (match + rest of string=w484:string)  [unwired: 1 in, 2 out]
          n287 = String Subset(string=w484, offset (0)=6 ("偏移量(0)"), length (rest)=6 ("长度（剩余）")) -> (substring=w481:string)
          n288 = case shown="\"w01019\"" w481 {
            tunnel: [0 ("长度（剩余）") 1 ("长度（剩余）") 2 ("长度（剩余）") 3 ("长度（剩余）") 4 ("长度（剩余）") 5 ("长度（剩余）")] -> w480
            frame "", Default {
            }
            frame "w01019" {
            }
            frame "w21003" {
            }
            frame "w21011" {
            }
            frame "w21001" {
            }
            frame "w01018" {
            }
          }
          n289 = Insert Into Array(array=u16[] [] ("holding register values"), index=0 ("索引"), new element=w480) -> (w485:u16[])
          n290 = case shown="\"3081\"" w479 {
            tunnel: [u16 99 ("starting address") u16 30 ("starting address") u16 31 ("starting address") u16 32 ("starting address") u16 33 ("starting address") u16 34 ("starting address") u16 35 ("starting address") u16 36 ("starting address")] -> w477
            frame "", Default {
            }
            frame "3080" {
            }
            frame "3081" {
            }
            frame "3082" {
            }
            frame "3083" {
            }
            frame "3084" {
            }
            frame "3085" {
            }
            frame "3086" {
            }
          }
          n291 = call "Modbus Master.vi"("Unit ID"=u8 1, "读取写入选择"="写入", "holding register values"=w485, "starting address"=w477) -> ()  [unwired: 6 in, 2 out]
        }
        frame #1 {
          n292 = Wait (ms)(milliseconds to wait=u32 3000 ("等待时间（毫秒）")) -> ()  [unwired: 1 out]
        }
        frame #2 {
          n293 = global write "全局1.vi" "table元素"("反控命令" ("新元素/子数组")) -> ()
          n294 = call "Modbus Master.vi"("Unit ID"=u8 1, "读取写入选择"="写入", "holding register values"=u16[] [0], "starting address"=w509) -> ("error out"=w506:errorcluster)  [unwired: 6 in, 1 out]
        }
        frame #3 {
        }
      }
    }
  }
  "反控命令错误？" <- w1
  n295 = case shown="假" w1 {
    tunnel: w2 -> [w513 _]
    frame False {
      n296 = global write "全局 反控命令枚举.vi" "是否判断反馈？"(w513) -> ()
    }
    frame True {
    }
  }
